vi "#5_old.vi"(0 "System no.":i32=1 min=1 max=4 step=1, 5 "error in":errorcluster) -> (14 "Overall system\nmoving?":bool, 15 "Sep. Axis 1\nmoving?":bool, 16 "Sep. Axis 2\nmoving?":bool, 19 "error out":errorcluster)   [LabVIEW 2020]
doc: "Polls the motion status of the F-206/M-8X0 and/or up to 2 additional connected axes by sending the single ASCII character 5. Required by General wait for movement to stop.vi.\n\nM-8X0: Only answer for overall system is valid."
panel:
  # "Polling-command for F-206 and M-850 (Sends Character 5 without\nLinefeed,  returns motion information for \nF-206 and up to 2 sep. stages   or   M-850)"
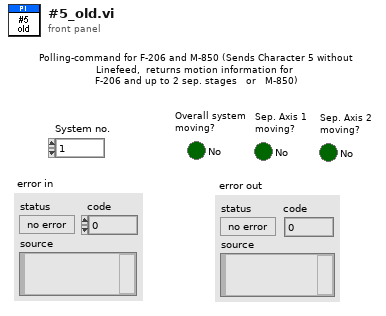
[diagram p1: front panel]
types:
  T1 = enum16{"Disable error check", "Force error check", "Use global settings"}
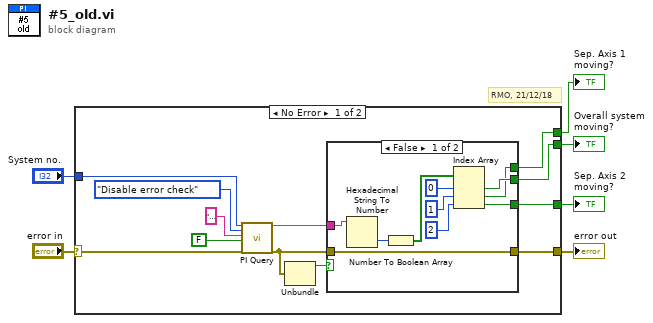
[diagram p0: block diagram]
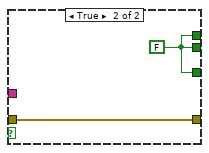
[diagram p2: hidden frame]
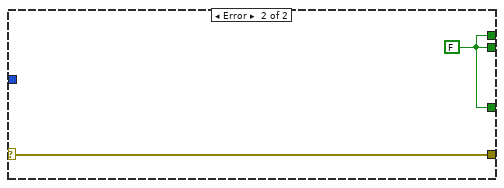
[diagram p3: hidden frame]
diagram:
  # "RMO, 21/12/18"
  n1 = case shown="No Error" "error in" {
    selector: "error in" -> [w7 w32]
    tunnel: [w15 w31] -> w6
    tunnel: [w14 w32] -> w5
    tunnel: [w13 w31] -> w4
    tunnel: [w12 w31] -> w3
    tunnel: "System no." -> [w11 _]
    frame No Error {
      n2 = call "PI Query.vi"("System no."=w11, "Error check settings"=T1."Disable error check", "String to send"="\u0005", "Attach termination char.?"=FALSE ("Attach Linefeed?"), "error in"=w7) -> ("String read"=w9:string, "error out"=w10:errorcluster)  [unwired: 2 in, 11 out]
      n3 = Unbundle(w10) -> ("status"=w16:bool)  [unwired: 2 out]
      n4 = case shown="False" w16 {
        tunnel: w9 -> [w22 _]
        tunnel: [w21 w29] -> w15
        tunnel: [w28 w30] -> w14
        tunnel: w10 -> [w28 w30]
        tunnel: [w20 w29] -> w13
        tunnel: [w19 w29] -> w12
        frame False {
          n5 = Hexadecimal String To Number(string=w22) -> (number=w27:u32)  [unwired: 3 out]
          n6 = Number To Boolean Array(number=w27) -> (Boolean array=w26:bool[])
          n7 = Index Array(array=w26, index #1=0 ("index"), index #2=1 ("index"), index #3=2 ("index")) -> (element #1=w21:bool, element #2=w20:bool, element #3=w19:bool)
        }
        frame True {
          w29 = FALSE
        }
      }
    }
    frame Error {
      w31 = FALSE
    }
  }
  "error out" <- w5
  "Overall system\nmoving?" <- w6
  "Sep. Axis 1\nmoving?" <- w4
  "Sep. Axis 2\nmoving?" <- w3
